vi "Write Execute Test VIs.vi"(8 "error in (no error)":errorcluster, 10 "Execute Test VIs":path[](array[path]), 11 "UnitTestEngine in":refnum<class "UnitTestEngine.lvclass">) -> (0 "error out":errorcluster, 3 "UnitTestEngine out":refnum<class "UnitTestEngine.lvclass">)   [LabVIEW 2019]
uses:
  UnitTestEngine.lvclass
  D:/TestBench/TestEngine/TestEngine/TestEngine.lvclass
  C:/Program Files (x86)/National Instruments/LabVIEW 2019/vi.lib/NI/Event Source Actor/Event Source/Event Source/Event Source.lvclass
  C:/Program Files (x86)/National Instruments/LabVIEW 2019/vi.lib/ActorFramework/Actor/Actor.lvclass
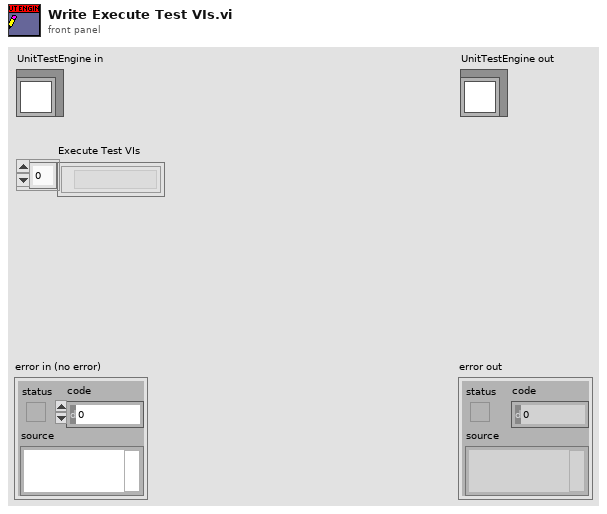
[diagram p1: front panel]
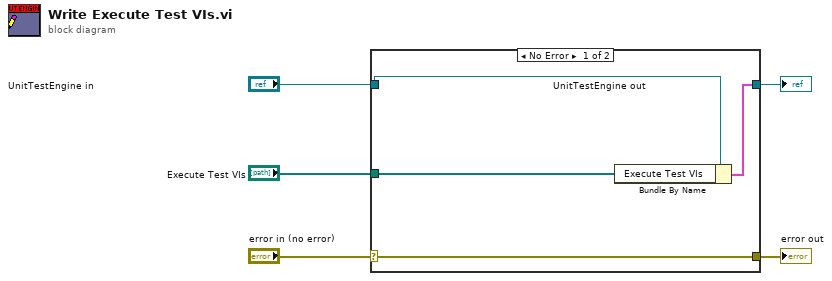
[diagram p0: block diagram]
diagram:
  n1 = case shown="No Error" "error in (no error)" {
    selector: "error in (no error)" -> [w9 w10]
    tunnel: [w9 w10] -> w4
    tunnel: [w7 w11] -> w2
    tunnel: "UnitTestEngine in" -> [w8 w11]
    tunnel: "Execute Test VIs" -> [w6 _]
    frame No Error {
      n2 = Bundle By Name(cluster=w8, "Execute Test VIs"=w6) -> (w7:cluster{})
    }
    frame Error {
    }
  }
  "error out" <- w4
  "UnitTestEngine out" <- w2
